vi "AddPathByQualifiedName.vi"(8 "error in (no error)":errorcluster, 9 "Path":string, 10 "Qualified name":string, 11 "CDependencyList in":refnum<class "CDependencyList.lvclass">) -> (0 "error out":errorcluster, 3 "CDependencyList out":refnum<class "CDependencyList.lvclass">)   [LabVIEW 2020, in "DependencyInspection.lvlib" / "CDependencyList.lvclass"]
uses:
  CDependencyList.lvclass
  CDependencyList.lvclass/CDependencyList.ctl
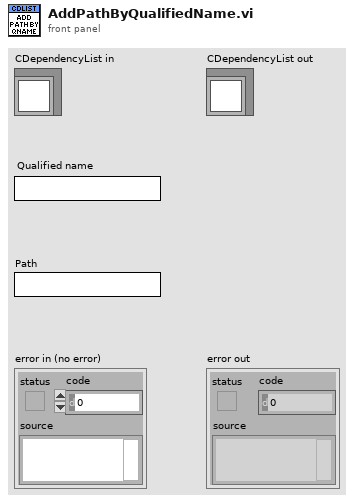
[diagram p1: front panel]
types:
  T1 = typedef "DependencyInspection.lvlib/CDependencyList.lvclass/QualifiedNamesToPathsMapRef.ctl" = refnum<data-value>
  T2 = typedef "DependencyInspection.lvlib/CDependencyList.lvclass/QualifiedNamesToPathsMap.ctl" = map{string, string}
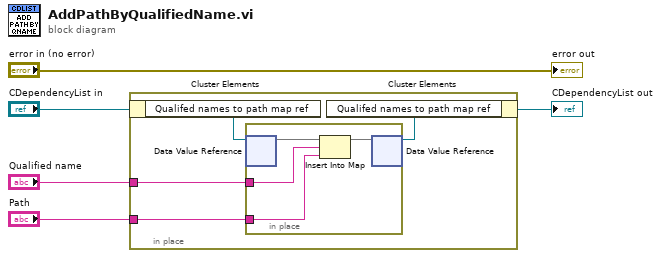
[diagram p0: block diagram]
diagram:
  n1 = in-place {
    in-place-border: "Qualified name" -> [w9]
    in-place-border: "Path" -> [w6]
    n2 = in-place-cluster #1("CDependencyList in") -> ("Qualifed names to path map ref"=w8:T1)
    n3 = in-place {
      in-place-border: w9 -> [w11]
      in-place-border: w6 -> [w10]
      n4 = in-place-dvr #2(w8) -> (w12:T2)  [unwired: 1 out]
      n5 = Insert Into Map(map in=w12, key=w11, value=w10) -> ()  [unwired: 3 out]
      n6 = in-place-dvr #2(w12) -> (w7:T1)  [unwired: 1 out]
    }
    n7 = in-place-cluster #1("Qualifed names to path map ref"=w7) -> (→"CDependencyList out":refnum<class "CDependencyList.lvclass">)
  }
  "error out" <- "error in (no error)"
